vi "Find Closest Tip to Point.vi"(8 "error in (no error)":errorcluster, 9 "Frame Number":i32, 10 "Point":T2 {"Y" format="%.2f"; "X" format="%.2f"}, 11 "Tips":T1[](array[typedef]) {"ROI Descriptor"."Contours"."Type" items=["No Selection", "Point", "Line", "Rectangle", "Oval", "Polygon", "Freehand Region", "Annulus", "Unused2", "Unused3", "Broken Line", "Freehand Line", "Rotated Rectangle"]; "Point"."Y" format="%.2f"; "Point"."X" format="%.2f"}) -> (0 "error out":errorcluster, 2 "Tip Index":i32, 3 "Tip":T1={"Point"={"X"=0.0, "Y"=0.0}, "Angle"=0.0, "Frame Number"=0, "ROI Descriptor"={"Global Rectangle"=[], "Contours"=[]}, "Curvature"=0.0, "Label"="Non-tip"} {"ROI Descriptor"."Contours"."Type" items=["No Selection", "Point", "Line", "Rectangle", "Oval", "Polygon", "Freehand Region", "Annulus", "Unused2", "Unused3", "Broken Line", "Freehand Line", "Rotated Rectangle"]; "Point"."Y" format="%.2f"; "Point"."X" format="%.2f"})   [LabVIEW 2013]
uses:
  Controls/Tip.ctl
  <vilib>/vision/NI_Vision_Development_Module.lvlib
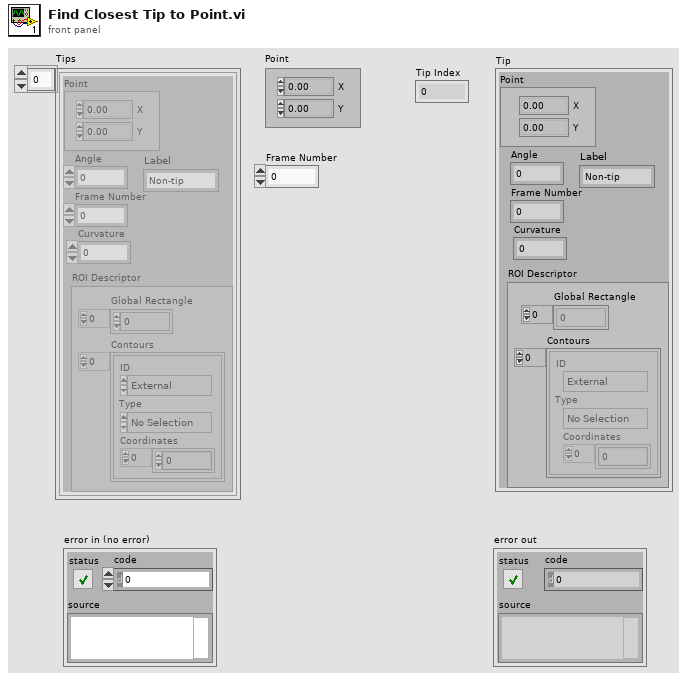
[diagram p1: front panel]
types:
  T1 = typedef "Tip.ctl" = cluster{"Point":T2, "Angle":dbl, "Frame Number":i32, "ROI Descriptor":T3, "Curvature":dbl, "Label":string}
  T2 = typedef "IMAQ Point" = cluster{"X":sgl, "Y":sgl}
  T3 = typedef "ROI Descriptor" = cluster{"Global Rectangle":i32[], "Contours":cluster{"ID":enum32{"External", "Internal"}, "Type":u32, "Coordinates":i32[]}[]}
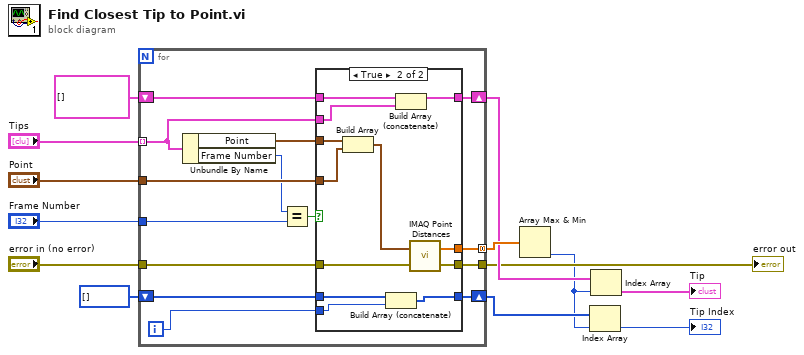
[diagram p0: block diagram]
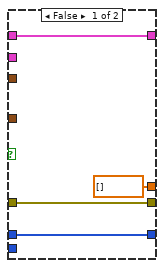
[diagram p2: hidden frame]
diagram:
  n1 = for {
    tunnel: "Tips" -> [w19] mode=indexing
    tunnel: "Point" -> [w26]
    tunnel: "error in (no error)" -> [w25]
    tunnel: [w24] -> w13 mode=concatenating
    tunnel: [w23] -> w8
    tunnel: "Frame Number" -> [w22]
    shift-right: [w17] -> w12
    shift-left: T1[] [] -> [w18]
    shift-right: [w14] -> w3
    shift-left: i32[] [] -> [w16]
    i -> [w15]
    n2 = Unbundle By Name(w19) -> ("Point"=w27:T2, "Frame Number"=w21:i32)
    n3 = Equal?(x=w21, y=w22) -> (x = y?=w20:bool)
    n4 = case shown="True" w20 {
      tunnel: w27 -> [_ w43]
      tunnel: w26 -> [_ w42]
      tunnel: w25 -> [w31 w41]
      tunnel: [sgl[] [] ("Distances") w39] -> w24
      tunnel: [w31 w38] -> w23
      tunnel: w19 -> [_ w37]
      tunnel: w18 -> [w29 w36]
      tunnel: [w29 w35] -> w17
      tunnel: w16 -> [w28 w34]
      tunnel: w15 -> [_ w33]
      tunnel: [w28 w32] -> w14
      frame False {
      }
      frame True {
        n5 = Build Array(w43, w42) -> (w40:T2[])
        n6 = Build Array (concatenate)(w34, w33) -> (w32:i32[])
        n7 = Build Array (concatenate)(w36, w37) -> (w35:T1[])
        n8 = call "IMAQ Point Distances"("Points"=w40, "error in (no error)"=w41) -> ("Distances"=w39:sgl[], "error out"=w38:errorcluster)  [unwired: 3 in]
      }
    }
  }
  "error out" <- w8
  n9 = Array Max & Min(array=w13) -> (min index (indices)=w2:i32)  [unwired: 3 out]
  n10 = Index Array(array=w3, index=w2) -> (element=→"Tip Index":i32)
  n11 = Index Array(array=w12, index=w2) -> (element=→"Tip":T1)
